vi "Events for UI Actor Indicators.vi"(6 "Mouse Position":T1, 7 "User VI Ref":refnum<vi>, 8 "Is Multi-select?":bool, 9 "Remaining Items":refnum<vi>[](array[refnum]), 10 "Affected Items":T8, 11 "Menu Refnum":refnum<k9>) -> (3 "Menu Items To Add":T2[](array[typedef]))   [LabVIEW 2020]
doc: "This VI is part of a plug-in for modifying the LabVIEW shortcut menus. This is the builder VI which is called when the shortcut menu is built. It tells LabVIEW which shortcut menu items to add to the menu."
uses:
  <resource>/plugins/PopupMenus/support/Shortcut Menu Item Definition.ctl
  <resource>/plugins/PopupMenus/support/Transaction Control.ctl
  <resource>/plugins/PopupMenus/support/Position In Menu.ctl
  <resource>/plugins/PopupMenus/support/Relative Position.ctl
  <resource>/plugins/PopupMenus/support/Checkmark Status.ctl
  <resource>/plugins/PopupMenus/support/Enabled Menu Item Status.ctl
  Events for UI Actor Indicators.ctl
  <vilib>/Utility/miscctls.llb/LVPositionTypeDef.ctl
  Events for UI Actor Indicators Support/Constants.vi
  <vilib>/UserTags/UserTags.lvlib
panel:
  # "Rules a popup plug-in must follow:\n* This VI's file name must match the file name of the LLB -- only the file extensions should be different.\n* This VI must have debugging disabled or it will be ignored as a plug-in.\n* For all menu items, \"tag suffix + file name of this VI\" must be less than 240 characters.\n* You can disconnect the \"Affected Items\" from the typedef to make the plug-in load faster. The typedef is only there to assist you in keeping this VI and the execution VI using to the same type.\n* All controls on this panel except \"Affected Items\" are locked to prevent accidental edits. Do not change the types or the names of controls other than the elements inside the \"Affected Items\" cluster.\n* See Context Help for more information on the individual controls."
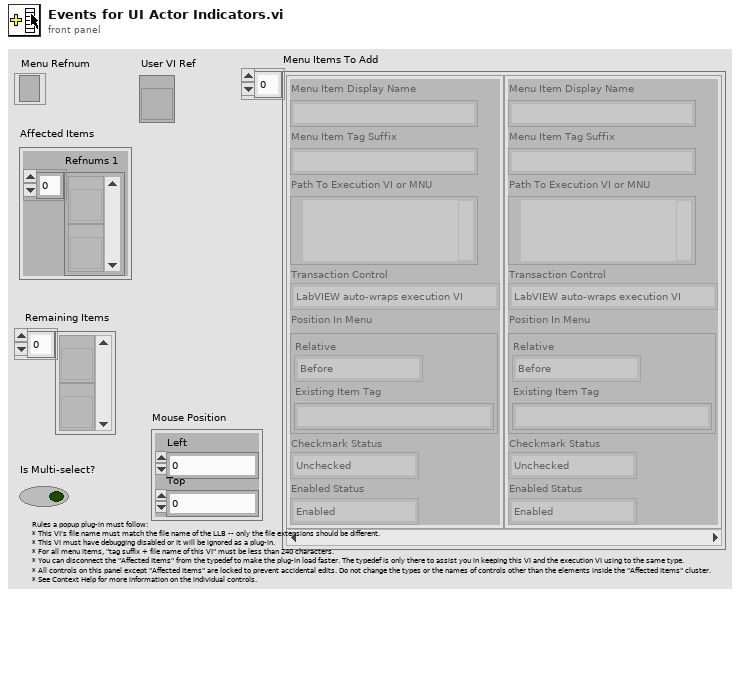
[diagram p1: front panel]
types:
  T1 = typedef "LVPositionTypeDef.ctl" = cluster{"Left":i32, "Top":i32}
  T2 = typedef "Shortcut Menu Item Definition.ctl" = cluster{"Menu Item Display Name":string, "Menu Item Tag Suffix":string, "Path To Execution VI or MNU":path, "Transaction Control":T3, "Position In Menu":T4, "Checkmark Status":T6, "Enabled Status":T7}
  T3 = typedef "Transaction Control.ctl" = enum8{"LabVIEW auto-wraps execution VI", "Execution VI will define if needed"}
  T4 = typedef "Position In Menu.ctl" = cluster{"Relative":T5, "Existing Item Tag":string}
  T5 = typedef "Relative Position.ctl" = enum8{"Before", "Instead of", "After", "Into Submenu"}
  T6 = typedef "Checkmark Status.ctl" = enum8{"Unchecked", "Checked"}
  T7 = typedef "Enabled Menu Item Status.ctl" = enum8{"Enabled", "Disabled"}
  T8 = typedef "Events for UI Actor Indicators.ctl" = cluster{"Refnums 1":refnum<vi>[]}
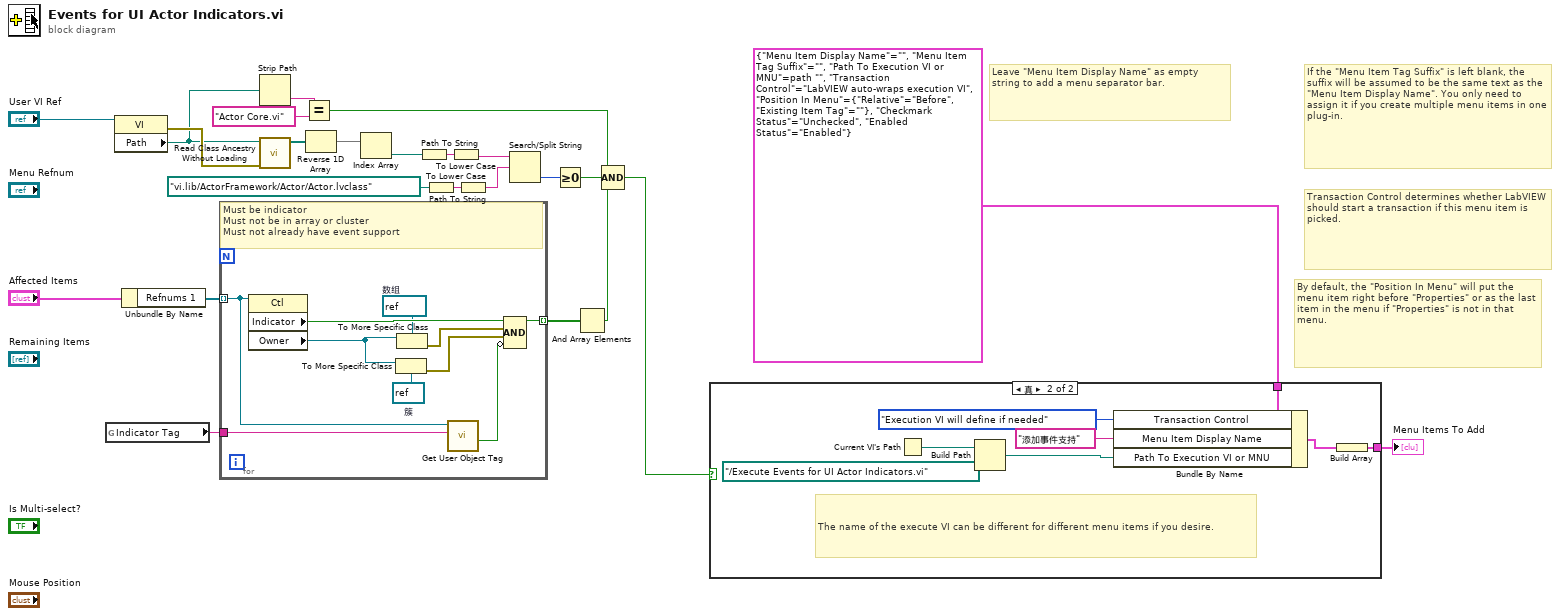
[diagram p0: block diagram]
diagram:
  # "Transaction Control determines whether LabVIEW should start a transaction if this menu item is picked."
  # "Leave \"Menu Item Display Name\" as empty string to add a menu separator bar."
  # "If the \"Menu Item Tag Suffix\" is left blank, the suffix will be assumed to be the same text as the \"Menu Item Display Name\". You only need to assign it if you create multiple menu items in one plug-in."
  # "By default, the \"Position In Menu\" will put the menu item right before \"Properties\" or as the last item in the menu if \"Properties\" is not in that menu."
  n1 = global read "Constants.vi" "Indicator Tag"() -> (w1:string)
  n2 = property class="VI"(reference="User VI Ref") -> (error out=w12:errorcluster, "Path"=w11:path)  [unwired: 1 in, 1 out]
  n3 = Unbundle By Name("Affected Items") -> ("Refnums 1"=w7:refnum<vi>[])
  n4 = for {
    tunnel: w7 -> [w30] mode=indexing
    tunnel: [w32] -> w6 mode=indexing
    tunnel: w1 -> [w25]
    w28 = refnum<vi> refnum  # 簇
    w33 = refnum<vi> refnum  # 数组
    # "Must be indicator\nMust not be in array or cluster\nMust not already have event support"
    n5 = property class="Ctl"(reference=w30) -> ("Indicator"=w34:bool, "Owner"=w27:refnum<vi>)  [unwired: 1 in, 2 out]
    n6 = To More Specific Class(target class=w28, reference=w27) -> (error out=w26:errorcluster)  [unwired: 1 in, 1 out]
    n7 = To More Specific Class(target class=w33, reference=w27) -> (error out=w31:errorcluster)  [unwired: 1 in, 1 out]
    n8 = call <vilib>:"Get User Object Tag.vi"("Tag Name"=w25, "Generic Refnum"=w30) -> ("Was Tag Found?"=w29:bool)  [unwired: 6 in, 3 out]
    n9 = Compound Arithmetic op=AND(w34, w31, w26, invert w29) -> (w32:bool)
  }
  n10 = Strip Path(path=w11) -> (name=w10:string)  [unwired: 1 out]
  n11 = call <vilib>:"Read Class Ancestry Without Loading.vi"("error in (no error)"=w12, "LabVIEW Class Path"=w11) -> ("Class Ancestry"=w20:path[])  [unwired: 8 in, 1 out]
  n12 = Equal?(x=w10, y="Actor Core.vi") -> (x = y?=w3:bool)
  n13 = Reverse 1D Array(array=w20) -> (reversed array=w19:path[])
  n14 = Index Array(array=w19) -> (element=w21:path)  [unwired: 1 in]
  n15 = Path To String(path=w21) -> (string=w17:string)
  n16 = Path To String(path=path "vi.lib/ActorFramework/Actor/Actor.lvclass") -> (string=w16:string)
  n17 = To Lower Case(string=w17) -> (all lower case string=w15:string)
  n18 = To Lower Case(string=w16) -> (all lower case string=w14:string)
  n19 = Search/Split String(string=w15, search string/char (-)=w14) -> (offset of match=w22:i32)  [unwired: 1 in, 2 out]
  n20 = Greater Or Equal To 0?(x=w22) -> (x >= 0?=w4:bool)
  n21 = And Array Elements(Boolean array=w6) -> (logical AND=w5:bool)
  n22 = Compound Arithmetic op=AND(w3, w4, w5) -> (w2:bool)
  n23 = case shown="真" w2 {
    tunnel: T2 {"Menu Item Display Name"="", "Menu Item Tag Suffix"="", "Path To Execution VI or MNU"=path "", "Transaction Control"=enum."LabVIEW auto-wraps execution VI", "Position In Menu"={"Relative"=enum."Before", "Existing Item Tag"=""}, "Checkmark Status"=enum."Unchecked", "Enabled Status"=enum."Enabled"} ("Cluster") -> [_ w40]
    tunnel: [_ w38] -> w23
    frame False {
    }
    frame True {
      # "The name of the execute VI can be different for different menu items if you desire."
      n24 = Current VI's Path() -> (path=w37:path)
      n25 = Build Path(base path=w37, name or relative path=path "../Execute Events for UI Actor Indicators.vi" ("execute path")) -> (appended path=w41:path)
      n26 = Bundle By Name(cluster=w40, "Transaction Control"=Transaction_Control."Execution VI will define if needed", "Menu Item Display Name"="添加事件支持", "Path To Execution VI or MNU"=w41) -> (w39:T2)
      n27 = Build Array(w39) -> (w38:T2[])
    }
  }
  "Menu Items To Add" <- w23
